vi "Read DIO Mode.vi"(8 "error in":errorcluster, 11 "Counter Driven Output Mode in":refnum<class "Counter Driven Output Mode.lvclass">) -> (0 "error out":errorcluster, 2 "DIO mode":u32, 3 "Counter Driven Output Mode out":refnum<class "Counter Driven Output Mode.lvclass">)   [LabVIEW 2017, in "Scan Engine Scripting.lvlib" / "Counter Driven Output Mode.lvclass"]
uses:
  Counter Driven Output Mode.lvclass
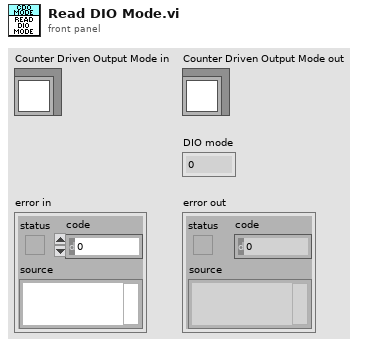
[diagram p1: front panel]
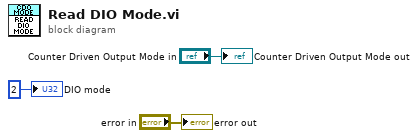
[diagram p0: block diagram]
diagram:
  "error out" <- "error in"
  "Counter Driven Output Mode out" <- "Counter Driven Output Mode in"
  "DIO mode" <- u32 2 ("DIO mode")
